vi "Get Map.vi"(10 "Project:Active Project":refnum<vi>) -> (2 "Type Name Path":map{string, map{string, path}}(c390))   [LabVIEW 2021, in "_Shared.lvlib"]
uses:
  _Shared.lvlib
  <vilib>/Nathan Davis/jettl/jettl/Queue/Queue.lvclass
  <vilib>/Nathan Davis/jettl/jettl/Event/Event.lvclass
  <vilib>/Nathan Davis/jettl/jettl/Msg Strategy/Msg Strategy.lvclass
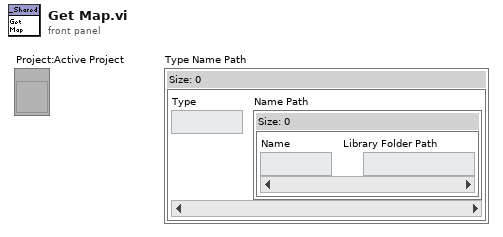
[diagram p1: front panel]
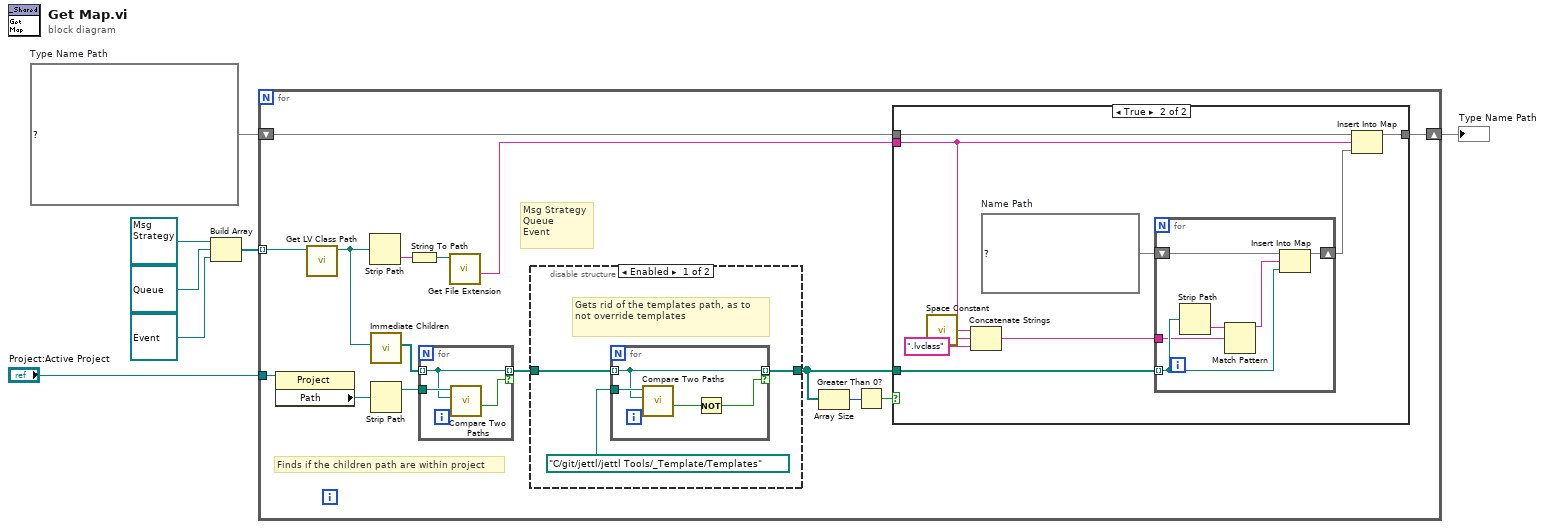
[diagram p0: block diagram]
diagram:
  w7 = map{string, map{string, path}} {}  # Type Name Path
  n1 = Build Array(refnum<class "Msg Strategy.lvclass"> refnum ("jettl.lvlib:Msg Strategy.lvclass"), refnum<class "Queue.lvclass"> refnum ("jettl.lvlib:Queue.lvclass"), refnum<class "Event.lvclass"> refnum ("jettl.lvlib:Event.lvclass")) -> (w3:refnum<class>[])
  n2 = for {
    shift-right: [w14] -> w2
    shift-left: w7 -> [w15]
    tunnel: w3 -> [w12] mode=indexing
    tunnel: "Project:Active Project" -> [w13]
    # "Msg Strategy\nQueue\nEvent"
    # "Finds if the children path are within project"
    n3 = property class="Project"(reference=w13) -> ("Path"=w22:path)  [unwired: 1 in, 2 out]
    n4 = call <vilib>:"Get LV Class Path.vi"("object"=w12) -> ("class path"=w8:path)  [unwired: 9 in, 1 out]
    n5 = Strip Path(path=w8) -> (name=w11:string)  [unwired: 1 out]
    n6 = call "Immediate Children.vi"("Path"=w8) -> ("Immediate Children Paths"=w19:path[])  [unwired: 9 in, 1 out]
    n7 = Strip Path(path=w22) -> (stripped path=w21:path)  [unwired: 1 out]
    n8 = String To Path(string=w11) -> (path=w10:path)
    n9 = for {
      tunnel: w19 -> [w47] mode=indexing
      tunnel: w21 -> [w48]
      tunnel: [w47] -> w20 mode=indexing if=w46
      n10 = call <vilib>:"Compare Two Paths.vi"("Path 2"=w47, "Path 1"=w48) -> ("Path 2 Relative to Path 1?"=w46:bool)  [unwired: 6 in, 3 out]
    }
    n11 = call <vilib>:"Get File Extension.vi"("file"=w10) -> ("filename without extension"=w9:string)  [unwired: 6 in, 4 out]
    n12 = disable-structure shown="Enabled" {
      disable-tunnel: w20 -> [w25 _]
      disable-tunnel: [w23 _] -> w17
      frame Enabled {
        # "Gets rid of the templates path, as to not override templates"
        n13 = for {
          tunnel: w25 -> [w28] mode=indexing
          tunnel: path "C:/git/jettl/jettl Tools/_Template/Templates" -> [w29]
          tunnel: [w28] -> w23 mode=indexing if=w26
          n14 = call <vilib>:"Compare Two Paths.vi"("Path 2"=w28, "Path 1"=w29) -> ("Path 2 Relative to Path 1?"=w27:bool)  [unwired: 6 in, 3 out]
          n15 = Not(x=w27) -> (.not. x?=w26:bool)
        }
      }
      frame Disabled {
      }
    }
    n16 = Array Size(array=w17) -> (size(s)=w18:i32)
    n17 = Greater Than 0?(x=w18) -> (x > 0?=w16:bool)
    n18 = case shown="True" w16 {
      tunnel: w17 -> [_ w39]
      tunnel: w9 -> [_ w31]
      tunnel: w15 -> [w30 w38]
      tunnel: [w30 w37] -> w14
      frame False {
      }
      frame True {
        w35 = map{string, path} {}  # Name Path
        n19 = call <vilib>:"Space Constant.vi"() -> ("String"=w33:string)
        n20 = Concatenate Strings(w33, w31, ".lvclass" ("string")) -> (w34:string)
        n21 = for {
          tunnel: w39 -> [w43] mode=indexing
          tunnel: w34 -> [w41]
          shift-right: [w44] -> w36
          shift-left: w35 -> [w45]
          n22 = Strip Path(path=w43) -> (name=w42:string)  [unwired: 1 out]
          n23 = Match Pattern(string=w42, regular expression=w41) -> (before substring=w40:string)  [unwired: 1 in, 3 out]
          n24 = Insert Into Map(map in=w45, key=w40, value=w43) -> (map out=w44:map{string, path})  [unwired: 2 out]
        }
        n25 = Insert Into Map(map in=w38, key=w31, value=w36) -> (map out=w37:map{string, map{string, path}})  [unwired: 2 out]
      }
    }
  }
  "Type Name Path" <- w2
